vi "Write file directory.vi"(8 "error in (no error)":errorcluster, 10 "file directory":path, 11 "current tag file io module configuration in":refnum<class "current tag file io module configuration.lvclass">) -> (0 "error out":errorcluster, 3 "current tag file io module configuration out":refnum<class "current tag file io module configuration.lvclass">)   [LabVIEW 2013]
uses:
  current tag file io module configuration.lvclass
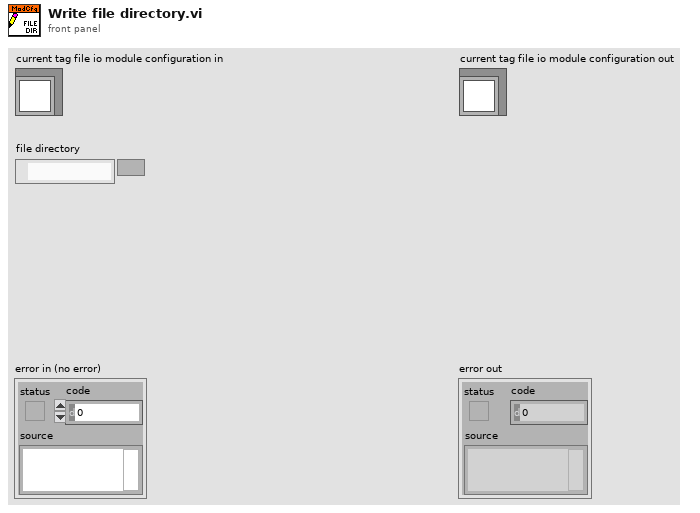
[diagram p1: front panel]
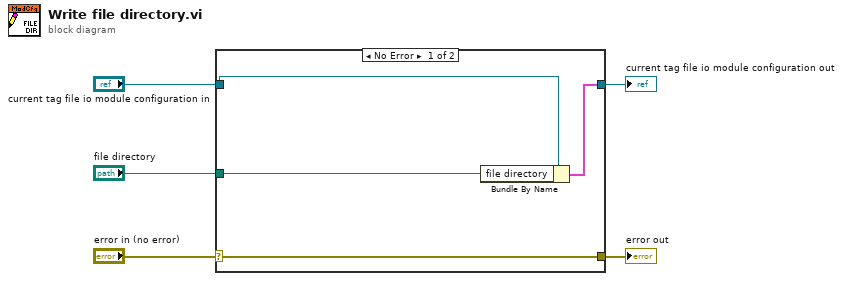
[diagram p0: block diagram]
diagram:
  n1 = case shown="No Error" "error in (no error)" {
    selector: "error in (no error)" -> [w9 w10]
    tunnel: [w9 w10] -> w4
    tunnel: [w7 w11] -> w2
    tunnel: "current tag file io module configuration in" -> [w8 w11]
    tunnel: "file directory" -> [w6 _]
    frame No Error {
      n2 = Bundle By Name(cluster=w8, "file directory"=w6) -> (w7:cluster{})
    }
    frame Error {
    }
  }
  "error out" <- w4
  "current tag file io module configuration out" <- w2
